vi "Interpolate 1D Fourier.vi"(6 "type":u16(ring)=1 items=["interpolation size", "interpolation factor"], 9 "dt in":dbl=1.0, 10 "n":i32=2, 11 "X":dbl[](array[numeric]) format="%_6g") -> (0 "error":i32, 1 "dt out":dbl, 2 "interpolation size":i32, 3 "Y":dbl[](array[numeric]) format="%_6g")   [LabVIEW 2017, in "NI_Gmath.lvlib"]
doc: "Performs interpolation by transforming the array <B>X</B> into the frequency domain, zero-padding and scaling appropriately for the interpolation factor you want and to maintain correct symmetry in the frequency domain, and then transforming back into the time domain to form the output interpolated array <B>Y out</B>."
uses:
  <vilib>/gmath/NI_Gmath.lvlib
  <vilib>/Analysis/2dsp.llb/Real FFT.vi
  <vilib>/Analysis/2dsp.llb/Inverse Real FFT.vi
  <vilib>/Analysis/NI_AALPro.lvlib
panel:
  # "Interpolate 1D\nFourier"
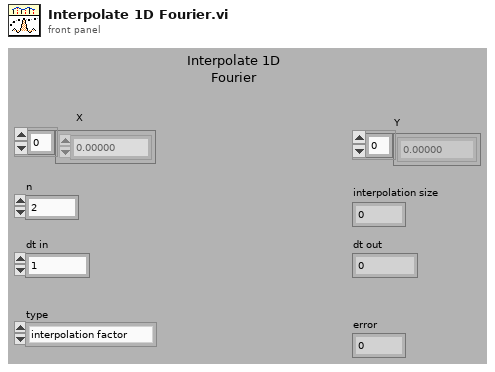
[diagram p1: front panel]
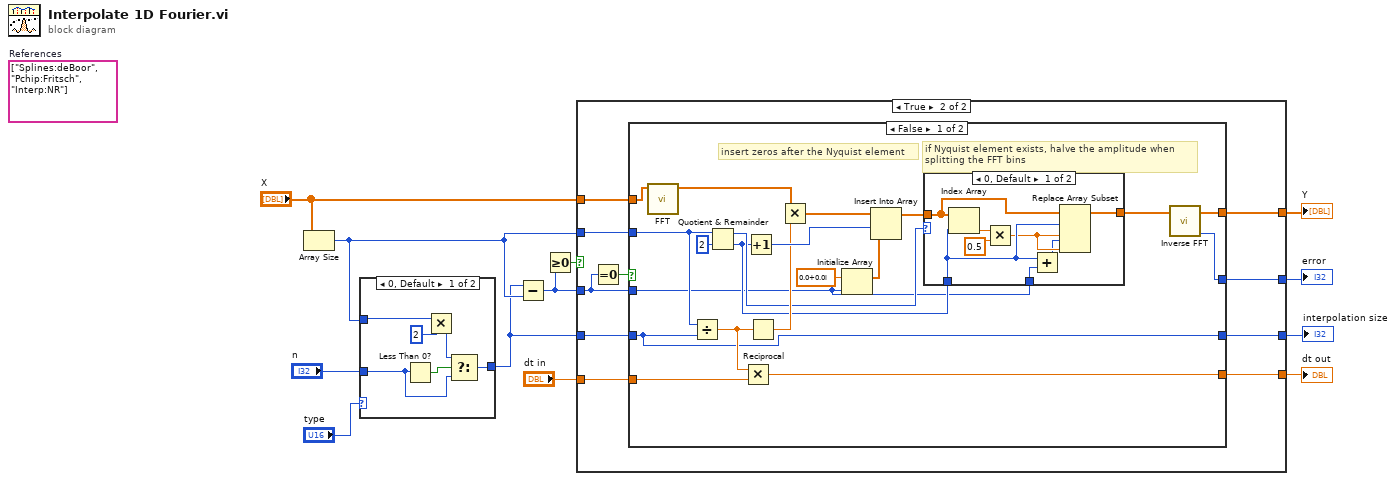
[diagram p0: block diagram]
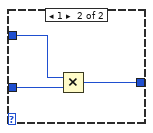
[diagram p2: hidden frame]
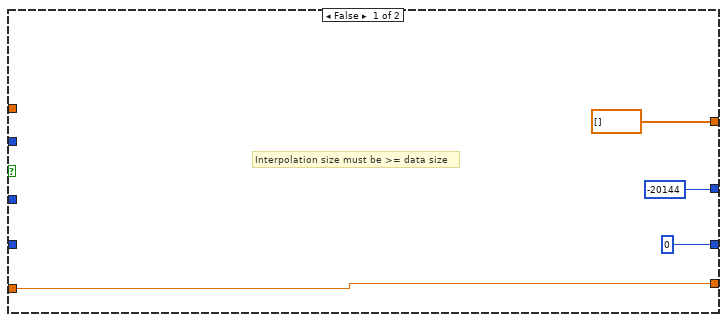
[diagram p3: hidden frame]
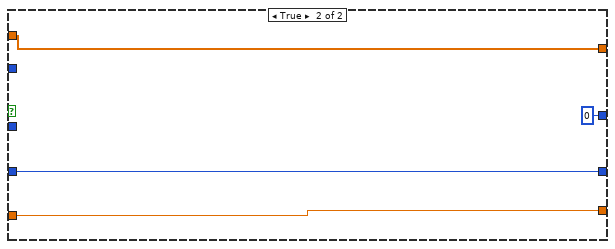
[diagram p5: hidden frame]
diagram:
  (unwired) string[] ["Splines:deBoor", "Pchip:Fritsch", "Interp:NR"]  # References
  n1 = Array Size(array="X") -> (size(s)=w5:i32)
  n2 = case shown="0, Default" "type" {
    tunnel: w5 -> [w16 w20]
    tunnel: "n" -> [w14 w21]
    tunnel: [w13 w19] -> w3
    frame 0, Default {
      n3 = Less Than 0?(x=w14) -> (x < 0?=w18:bool)
      n4 = Multiply(x=w16, y=2) -> (x*y=w15:i32)
      n5 = Select(t=w15, s=w18, f=w14) -> (s? t:f=w13:i32)
    }
    frame 1 {
      n6 = Multiply(x=w20, y=w21) -> (x*y=w19:i32)
    }
  }
  n7 = Subtract(x=w3, y=w5) -> (x-y=w6:i32)
  n8 = Greater Or Equal To 0?(x=w6) -> (x >= 0?=w12:bool)
  n9 = case shown="True" w12 {
    tunnel: [-20144 ("n") w29] -> w11
    tunnel: "X" -> [_ w35]
    tunnel: [dbl[] [] ("Y") w34] -> w9
    tunnel: "dt in" -> [w24 w31]
    tunnel: [w24 w30] -> w7
    tunnel: w5 -> [_ w33]
    tunnel: w3 -> [_ w32]
    tunnel: w6 -> [_ w27]
    tunnel: [0 ("n") w26] -> w1
    frame False {
      # "Interpolation size must be >= data size"
    }
    frame True {
      n10 = Equal To 0?(x=w27) -> (x = 0?=w28:bool)
      n11 = case shown="False" w28 {
        tunnel: w35 -> [w55 w68]
        tunnel: [w50 w68] -> w34
        tunnel: w33 -> [w49 _]
        tunnel: w32 -> [w37 w65]
        tunnel: w31 -> [w48 w67]
        tunnel: [w36 w67] -> w30
        tunnel: [w39 0 ("error")] -> w29
        tunnel: w27 -> [w38 _]
        tunnel: [w37 w65] -> w26
        frame False {
          # "if Nyquist element exists, halve the amplitude when\nsplitting the FFT bins"
          # "insert zeros after the Nyquist element"
          n12 = call-poly <vilib>:"FFT.vi"("X"=w55) -> ("FFT {X}"=w47:cdb[])  [unwired: 9 in, 1 out]
          n13 = Divide(x=w49, y=w37) -> (x/y=w44:dbl)
          n14 = Quotient & Remainder(x=w49, y=2) -> (x-y*floor(x/y)=w42:i32, floor(x/y)=w41:i32)
          n15 = Multiply(x=w44, y=w48) -> (x*y=w36:dbl)
          n16 = Increment(x=w41) -> (x+1=w52:i32)
          n17 = Reciprocal(x=w44) -> (1/x=w46:dbl)
          n18 = Multiply(x=w47, y=w46) -> (x*y=w45:cdb[])
          n19 = Initialize Array(cdb 0.0+0.0i ("element"), w38) -> (w51:cdb[])
          n20 = Insert Into Array(array=w45, index=w52, new element=w51) -> (w43:cdb[])
          n21 = case shown="0, Default" w42 {
            tunnel: w43 -> [w61 w64]
            tunnel: w41 -> [w60 _]
            tunnel: [w58 w64] -> w40
            tunnel: w38 -> [w59 _]
            frame 0, Default {
              n22 = Index Array(array=w61, index=w60) -> (element=w63:cdb)
              n23 = Multiply(x=w63, y=0.5) -> (x*y=w57:cdb)
              n24 = Add(x=w60, y=w59) -> (x+y=w56:i32)
              n25 = Replace Array Subset(array=w61, new element #1=w57, index #1=w60, new element #2=w57, index #2=w56) -> (w58:cdb[])
            }
            frame 1 {
            }
          }
          n26 = call-poly <vilib>:"Inverse FFT.vi"("FFT {X}"=w40) -> ("error"=w39:i32, "X"=w50:dbl[])  [unwired: 9 in]
        }
        frame True {
        }
      }
    }
  }
  "Y" <- w9
  "error" <- w11
  "dt out" <- w7
  "interpolation size" <- w1
